vi "get_shooter_commands.vi"(11 "Driver Inputs":T1) -> (3 "Circular Shooter Commands":T3)   [LabVIEW 2012]
uses:
  circular_shooter_commands.ctl
  Joystick_Inputs.ctl
  <vilib>/Rock Robotics/WPI/Joystick/WPI_JoystickButtonState.ctl
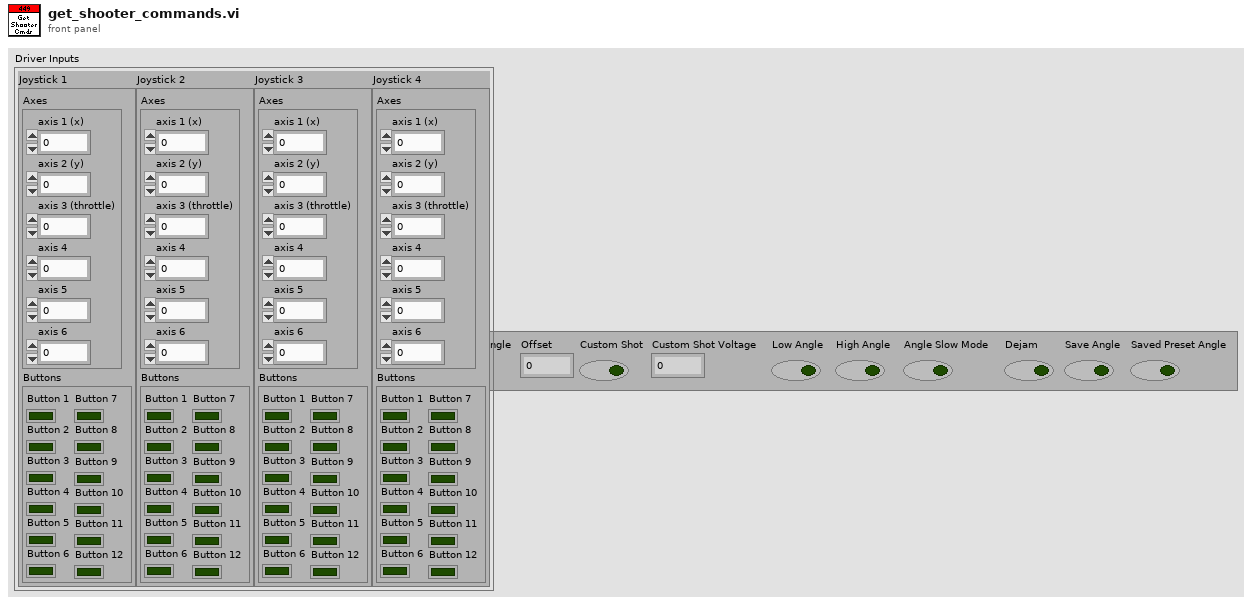
[diagram p1: front panel]
types:
  T1 = typedef "Joystick_Inputs.ctl" = cluster{"Joystick 1":cluster{"Axes":cluster{"axis 1 (x)":dbl, "axis 2 (y)":dbl, "axis 3 (throttle)":dbl, "axis 4":dbl, "axis 5":dbl, "axis 6":dbl}, "Buttons":T2}, "Joystick 2":cluster{"Axes":cluster{"axis 1 (x)":dbl, "axis 2 (y)":dbl, "axis 3 (throttle)":dbl, "axis 4":dbl, "axis 5":dbl, "axis 6":dbl}, "Buttons":T2}, "Joystick 3":cluster{"Axes":cluster{"axis 1 (x)":dbl, "axis 2 (y)":dbl, "axis 3 (throttle)":dbl, "axis 4":dbl, "axis 5":dbl, "axis 6":dbl}, "Buttons":T2}, "Joystick 4":cluster{"Axes":cluster{"axis 1 (x)":dbl, "axis 2 (y)":dbl, "axis 3 (throttle)":dbl, "axis 4":dbl, "axis 5":dbl, "axis 6":dbl}, "Buttons":T2}}
  T2 = typedef "WPI_JoystickButtonState.ctl" = cluster{"Button 1":bool, "Button 2":bool, "Button 3":bool, "Button 4":bool, "Button 5":bool, "Button 6":bool, "Button 7":bool, "Button 8":bool, "Button 9":bool, "Button 10":bool, "Button 11":bool, "Button 12":bool}
  T3 = typedef "circular_shooter_commands.ctl" = cluster{"Shoot?":bool, "Angle Change":dbl, "Close Shot":bool, "Far Shot":bool, "Stabilize Angle ":bool, "Offset":dbl, "Custom Shot":bool, "Custom Shot Voltage":dbl, "Low Angle":bool, "High Angle":bool, "Angle Slow Mode":bool, "Dejam":bool, "Save Angle":bool, "Saved Preset Angle":bool}
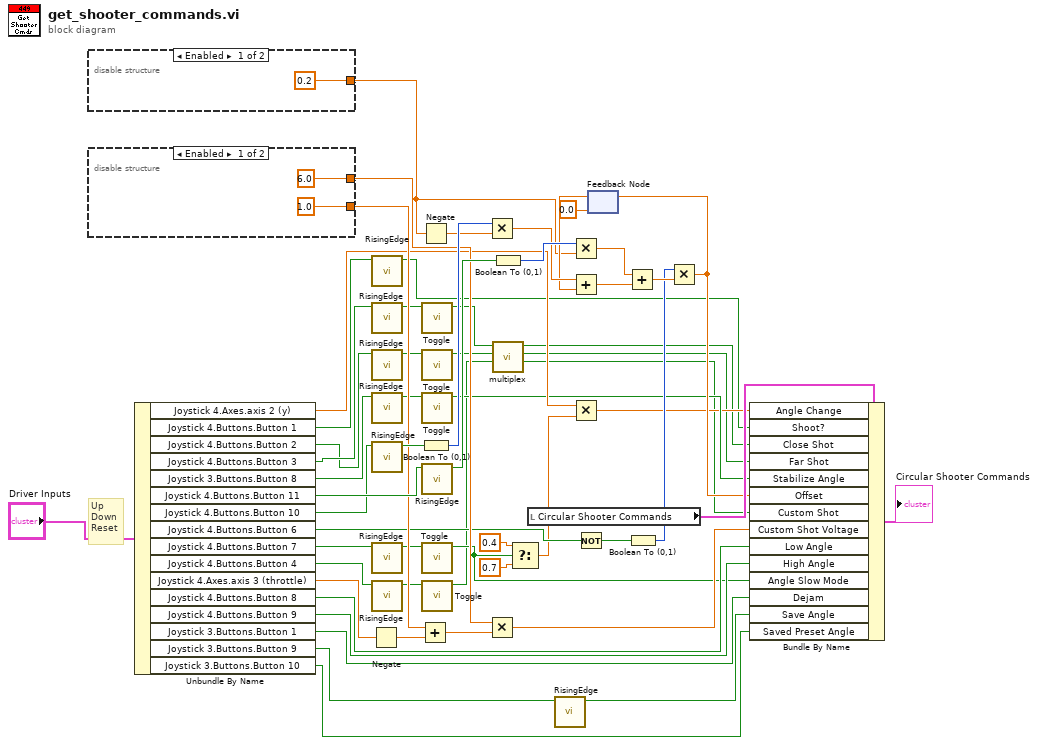
[diagram p0: block diagram]
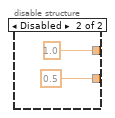
[diagram p2: hidden frame]
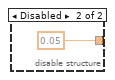
[diagram p3: hidden frame]
diagram:
  # "Up\nDown\nReset"
  n1 = disable-structure shown="Enabled" {
    disable-tunnel: [0.2 0.05] -> w7
    frame Enabled {
    }
    frame Disabled {
    }
  }
  n2 = disable-structure shown="Enabled" {
    disable-tunnel: [6.0 ("x") 1.0 ("x")] -> w36
    disable-tunnel: [1.0 0.5] -> w33
    frame Enabled {
    }
    frame Disabled {
    }
  }
  n3 = Unbundle By Name("Driver Inputs") -> ("Joystick 4.Axes.axis 2 (y)"=w32:dbl, "Joystick 4.Buttons.Button 1"=w56:bool, "Joystick 4.Buttons.Button 2"=w2:bool, "Joystick 4.Buttons.Button 3"=w3:bool, "Joystick 3.Buttons.Button 8"=w54:bool, "Joystick 4.Buttons.Button 11"=w52:bool, "Joystick 4.Buttons.Button 10"=w51:bool, "Joystick 4.Buttons.Button 6"=w26:bool, "Joystick 4.Buttons.Button 7"=w21:bool, "Joystick 4.Buttons.Button 4"=w15:bool, "Joystick 4.Axes.axis 3 (throttle)"=w38:dbl, "Joystick 4.Buttons.Button 8"=w28:bool, "Joystick 4.Buttons.Button 9"=w27:bool, "Joystick 3.Buttons.Button 1"=w1:bool, "Joystick 3.Buttons.Button 9"=w6:bool, "Joystick 3.Buttons.Button 10"=w4:bool)
  n4 = Negate(x=w38) -> (-x=w31:dbl)
  n5 = call "RisingEdge.vi"("BooleanIn"=w56) -> ("BooleanOut"=w17:bool)  [unwired: 10 in]
  n6 = call "RisingEdge.vi"("BooleanIn"=w3) -> ("BooleanOut"=w16:bool)  [unwired: 10 in]
  n7 = call "RisingEdge.vi"("BooleanIn"=w2) -> ("BooleanOut"=w18:bool)  [unwired: 10 in]
  n8 = call "RisingEdge.vi"("BooleanIn"=w54) -> ("BooleanOut"=w29:bool)  [unwired: 10 in]
  n9 = call "RisingEdge.vi"("BooleanIn"=w51) -> ("BooleanOut"=w34:bool)  [unwired: 10 in]
  n10 = call "RisingEdge.vi"("BooleanIn"=w21) -> ("BooleanOut"=w20:bool)  [unwired: 10 in]
  n11 = call "RisingEdge.vi"("BooleanIn"=w15) -> ("BooleanOut"=w14:bool)  [unwired: 10 in]
  n12 = Add(x=w33, y=w31) -> (x+y=w37:dbl)
  n13 = Negate(x=w7) -> (-x=w47:dbl)
  n14 = Boolean To (0,1)(Boolean=w34) -> (0, 1=w48:i16)
  n15 = call "Toggle.vi"("Toggle"=w16) -> ("BoolOut"=w13:bool)  [unwired: 10 in]
  n16 = call "Toggle.vi"("Toggle"=w18) -> ("BoolOut"=w12:bool)  [unwired: 10 in]
  n17 = call "Toggle.vi"("Toggle"=w29) -> ("BoolOut"=w30:bool)  [unwired: 10 in]
  n18 = call "RisingEdge.vi"("BooleanIn"=w52) -> ("BooleanOut"=w50:bool)  [unwired: 10 in]
  n19 = call "Toggle.vi"("Toggle"=w20) -> ("BoolOut"=w19:bool)  [unwired: 10 in]
  n20 = call "Toggle.vi"("Toggle"=w14) -> ("BoolOut"=w11:bool)  [unwired: 10 in]
  n21 = Multiply(x=w48, y=w47) -> (x*y=w46:dbl)
  n22 = Multiply(x=w36, y=w37) -> (x*y=w35:dbl)
  n23 = Boolean To (0,1)(Boolean=w50) -> (0, 1=w49:i16)
  n24 = call "multiplex.vi"("in 3"=w11, "in 2"=w12, "in 1"=w13) -> ("out 3"=w8:bool, "out 2"=w9:bool, "out 1"=w10:bool)  [unwired: 6 in]
  n25 = Select(t=0.4, s=w19, f=0.7) -> (s? t:f=w22:dbl)
  n26 = local read "Circular Shooter Commands"() -> (w57:T3)
  n27 = call "RisingEdge.vi"("BooleanIn"=w6) -> ("BooleanOut"=w5:bool)  [unwired: 10 in]
  n28 = Multiply(x=w49, y=w7) -> (x*y=w44:dbl)
  n29 = Multiply(x=w32, y=w22) -> (x*y=w23:dbl)
  n30 = Not(x=w26) -> (.not. x?=w41:bool)
  n31 = feedback #1(0.0) -> (w45:dbl)
  n32 = Add(x=w46, y=w45) -> (x+y=w43:dbl)
  n33 = Add(x=w44, y=w43) -> (x+y=w42:dbl)
  n34 = Boolean To (0,1)(Boolean=w41) -> (0, 1=w39:i16)
  n35 = Multiply(x=w39, y=w42) -> (x*y=w40:dbl)
  n36 = feedback-in #1(w40) -> ()
  n37 = Bundle By Name(cluster=w57, "Angle Change"=w23, "Shoot?"=w17, "Close Shot"=w10, "Far Shot"=w9, "Stabilize Angle"=w30, "Offset"=w40, "Custom Shot"=w8, "Custom Shot Voltage"=w35, "Low Angle"=w28, "High Angle"=w27, "Angle Slow Mode"=w19, "Dejam"=w1, "Save Angle"=w5, "Saved Preset Angle"=w4) -> (→"Circular Shooter Commands":T3)
